vi "Release Notifier.vi"(8 "error in":errorcluster, 11 "NotifierMessageTransport in":refnum<class "NotifierMessageTransport.lvclass">) -> (0 "error out":errorcluster, 3 "NotifierMessageTransport out":refnum<class "NotifierMessageTransport.lvclass">)   [LabVIEW 2016, in "NotifierMessageTransport.lvclass"]
uses:
  NotifierMessageTransport.lvclass
  NotifierMessageTransport.lvclass/NotifierMessageTransport.ctl
  IMessagePayload/IMessagePayload.lvclass
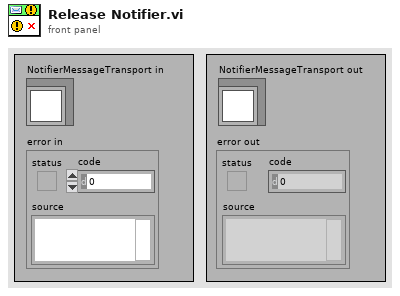
[diagram p1: front panel]
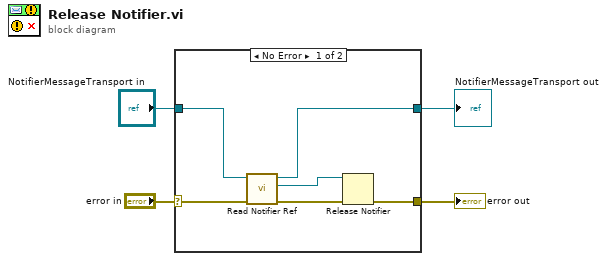
[diagram p0: block diagram]
diagram:
  n1 = case shown="No Error" "error in" {
    selector: "error in" -> [w10 w12]
    tunnel: [w5 w12] -> w3
    tunnel: [w6 w11] -> w1
    tunnel: "NotifierMessageTransport in" -> [w7 w11]
    frame No Error {
      n2 = call "Read Notifier Ref.vi"("error in"=w10, "NotifierMessageTransport in"=w7) -> ("error out"=w9:errorcluster, "Notifier Ref"=w8:refnum<notifier>, "NotifierMessageTransport out"=w6:refnum<class "NotifierMessageTransport.lvclass">)  [unwired: 7 in]
      n3 = Release Notifier(notifier=w8, error in (no error)=w9) -> (error out=w5:errorcluster)  [unwired: 1 in, 2 out]
    }
    frame Error {
    }
  }
  "error out" <- w3
  "NotifierMessageTransport out" <- w1
